vi "GoTo Tangent.vi"(8 "Target to kick":dbl[](array[numeric]), 9 "Ball":dbl[](array[numeric]), 10 "R (sem orientação)":dbl[](array[numeric]), 11 "R (com orientação)":dbl[](array[numeric])) -> (2 "Output\nVelocity":dbl[](array[numeric]) format="%.2f")   [LabVIEW 2016]
panel:
  in  "distance between ball and robot":dbl=200.0 format="%#_13g"
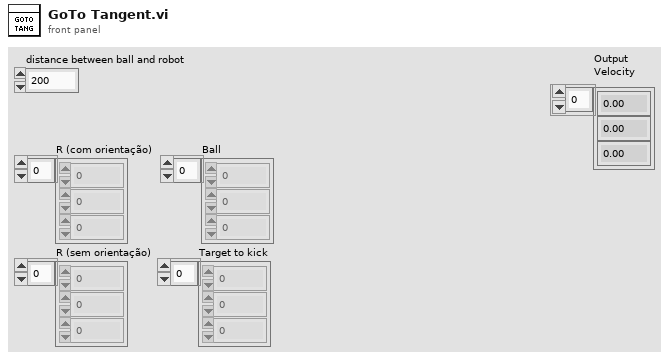
[diagram p1: front panel]
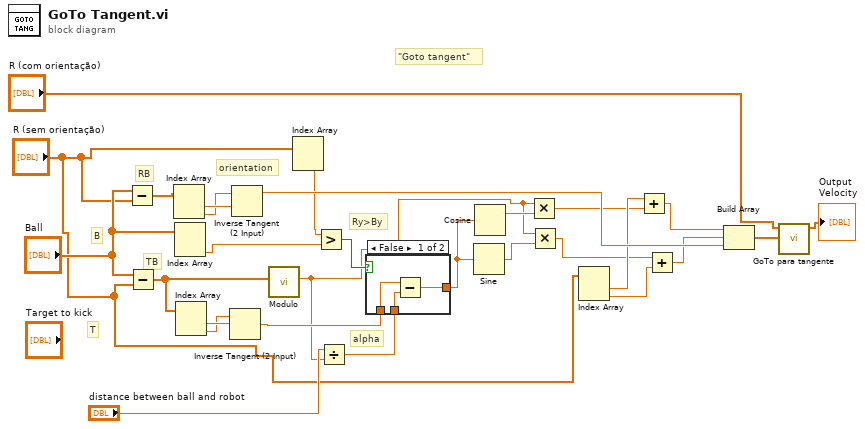
[diagram p0: block diagram]
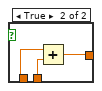
[diagram p2: hidden frame]
diagram:
  # "\"Goto tangent\""
  # "Ry>By"
  # "orientation"
  # "RB"
  # "alpha"
  # "TB"
  # "B"
  # "T"
  n1 = Subtract(x="Ball", y="R (sem orientação)") -> (x-y=w22:dbl[])
  n2 = Subtract(x="Ball", y="R (sem orientação)") -> (x-y=w26:dbl[])
  n3 = Index Array(array=w22) -> (element #1=w24:dbl, element #2=w23:dbl)  [unwired: 2 in]
  n4 = Index Array(array="Ball") -> (element #2=w14:dbl)  [unwired: 2 in, 1 out]
  n5 = Index Array(array=w26) -> (element #1=w28:dbl, element #2=w27:dbl)  [unwired: 2 in]
  n6 = Inverse Tangent (2 Input)(1:w28, 2:w27) -> (0:w20:dbl)
  n7 = Inverse Tangent (2 Input)(1:w24, 2:w23) -> (0:w21:dbl)
  n8 = call "Modulo.vi"("2D vector"=w26) -> ("Modulo"=w12:dbl)  [unwired: 10 in]
  n9 = Index Array(array="R (sem orientação)") -> (element #2=w15:dbl)  [unwired: 2 in, 1 out]
  n10 = Greater?(x=w15, y=w14) -> (0:w13:bool)
  n11 = Divide(x="distance between ball and robot", y=w12) -> (x/y=w19:dbl)
  n12 = case shown="False" w13 {
    tunnel: w20 -> [w30 w34]
    tunnel: w19 -> [w31 w33]
    tunnel: [w29 w32] -> w18
    frame False {
      n13 = Subtract(x=w30, y=w31) -> (x-y=w29:dbl)
    }
    frame True {
      n14 = Add(x=w34, y=w33) -> (x+y=w32:dbl)
    }
  }
  n15 = Sine(x=w18) -> (sin(x)=w16:dbl)
  n16 = Cosine(x=w18) -> (cos(x)=w17:dbl)
  n17 = Multiply(x=w12, y=w17) -> (x*y=w10:dbl)
  n18 = Multiply(x=w12, y=w16) -> (x*y=w6:dbl)
  n19 = Index Array(array="R (sem orientação)") -> (element #1=w11:dbl, element #2=w5:dbl)  [unwired: 2 in]
  n20 = Add(x=w11, y=w10) -> (x+y=w9:dbl)
  n21 = Add(x=w6, y=w5) -> (x+y=w4:dbl)
  n22 = Build Array(w9, w4, w21) -> (w1:dbl[])
  n23 = call "GoTo para tangente.vi"("Target"=w1, "Position"="R (com orientação)") -> ("Output\nVelocity"=→"Output\nVelocity":dbl[])  [unwired: 8 in, 1 out]
